vi "Untitled 1.vi"   [LabVIEW 2014]
uses:
  <vilib>/Rock Robotics/WPI/Solenoid/WPI_SolenoidValue.ctl
  <vilib>/Rock Robotics/WPI/Solenoid/WPI_SolenoidSetEnum.vi
  Robot Global Data.vi
types:
  T1 = typedef "WPI_SolenoidValue.ctl" = enum16{"Off", "On", "Forward", "Reverse"}
  T2 = typedef "WPI_SolenoidDevRef.ctl" = cluster{"DevStatus":errorcluster, "Pneumatics Control Module":u8, "Forward Solenoid Channel":T3, "Reverse Solenoid Channel":T3}
  T3 = typedef "WPI_SolenoidChannel.ctl" = enum8{"Solenoid 0", "Solenoid 1", "Solenoid 2", "Solenoid 3", "Solenoid 4", "Solenoid 5", "Solenoid 6", "Solenoid 7", "Invalid"}
  T4 = typedef "WPI_EncoderDevRef.ctl" = cluster{"DevStatus":errorcluster, "EncoderIndex":T5, "CounterIndex":T6, "DistancePerCount":dbl, "Decoding Type":T7}
  T5 = typedef "FPGA_EncoderIdx.ctl" = enum8{"Enc 0", "Enc 1", "Enc 2", "Enc 3", "Enc 4", "Enc 5", "Enc 6", "Enc 7", "Invalid"}
  T6 = typedef "FPGA_CounterCtrSystemIndex.ctl" = enum8{"Ctr 0", "Ctr 1", "Ctr 2", "Ctr 3", "Ctr 4", "Ctr 5", "Ctr 6", "Ctr 7", "Invalid"}
  T7 = typedef "WPI_EncoderType.ctl" = enum16{"1x", "2x", "4x"}
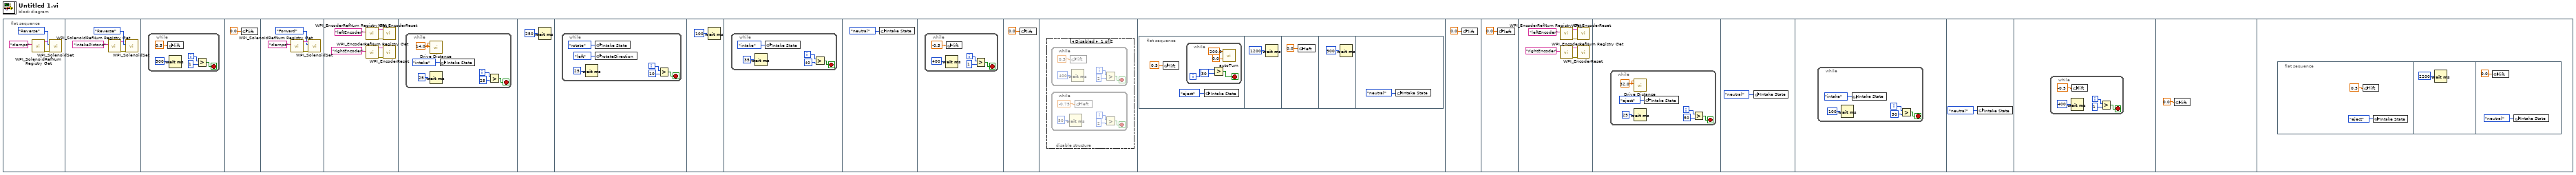
[diagram p0: block diagram]
diagram:
  n1 = flat-sequence {
    frame #0 {
      n2 = call <vilib>:"WPI_SolenoidRefNum Registry Get.vi"("refnum name"="clamps") -> ("error out"=w1:errorcluster, "SolenoidDevRef"=w2:T2)  [unwired: 9 in]
      n3 = call-poly <vilib>:"WPI_SolenoidSet.vi"("error in (no error)"=w1, "Value"=WPI_SolenoidValue."Reverse", "SolenoidDevRef"=w2) -> ()  [unwired: 7 in, 2 out]
    }
    frame #1 {
      n4 = call <vilib>:"WPI_SolenoidRefNum Registry Get.vi"("refnum name"="intakePistons") -> ("error out"=w5:errorcluster, "SolenoidDevRef"=w6:T2)  [unwired: 9 in]
      n5 = call-poly <vilib>:"WPI_SolenoidSet.vi"("error in (no error)"=w5, "Value"=WPI_SolenoidValue."Reverse", "SolenoidDevRef"=w6) -> ()  [unwired: 7 in, 2 out]
    }
    frame #2 {
      n6 = while {
        i -> [w11]
        stop <- w9 stop-if-true
        n7 = global write "Robot Global Data.vi" "lift"(0.5 ("lift")) -> ()
        n8 = Wait (ms)(milliseconds to wait=u32 500) -> ()  [unwired: 1 out]
        n9 = Greater?(x=w11, y=1) -> (0:w9:bool)
      }
    }
    frame #3 {
      n10 = global write "Robot Global Data.vi" "lift"(0.0 ("lift")) -> ()
    }
    frame #4 {
      n11 = call <vilib>:"WPI_SolenoidRefNum Registry Get.vi"("refnum name"="clamps") -> ("error out"=w18:errorcluster, "SolenoidDevRef"=w17:T2)  [unwired: 9 in]
      n12 = call-poly <vilib>:"WPI_SolenoidSet.vi"("error in (no error)"=w18, "Value"=WPI_SolenoidValue."Forward", "SolenoidDevRef"=w17) -> ()  [unwired: 7 in, 2 out]
    }
    frame #5 {
      n13 = call <vilib>:"WPI_EncoderRefNum Registry Get.vi"("refnum name"="leftEncoder") -> ("error out"=w24:errorcluster, "EncoderDevRef"=w23:T4)  [unwired: 9 in]
      n14 = call <vilib>:"WPI_EncoderRefNum Registry Get.vi"("refnum name"="rightEncoder") -> ("error out"=w19:errorcluster, "EncoderDevRef"=w20:T4)  [unwired: 9 in]
      n15 = call <vilib>:"WPI_EncoderReset.vi"("error in (no error)"=w24, "EncoderDevRef"=w23) -> ()  [unwired: 8 in, 2 out]
      n16 = call <vilib>:"WPI_EncoderReset.vi"("error in (no error)"=w19, "EncoderDevRef"=w20) -> ()  [unwired: 8 in, 2 out]
    }
    frame #6 {
      n17 = while {
        i -> [w28]
        stop <- w26 stop-if-true
        w29 = 14.0 ("Desired Right Inches")
        n18 = call "Drive Distance.vi"("Desired Right Inches"=w29, "Desired Left Inches"=w29) -> ()  [unwired: 10 in]
        n19 = Wait (ms)(milliseconds to wait=u32 25) -> ()  [unwired: 1 out]
        n20 = global write "Robot Global Data.vi" "Intake State"(enum16{"neutral", "rotate", "intake", "eject"}."intake" ("Intake State")) -> ()
        n21 = Greater?(x=w28, y=25) -> (0:w26:bool)
      }
    }
    frame #7 {
      n22 = Wait (ms)(milliseconds to wait=u32 250) -> ()  [unwired: 1 out]
    }
    frame #8 {
      n23 = while {
        i -> [w35]
        stop <- w34 stop-if-true
        n24 = Wait (ms)(milliseconds to wait=u32 25) -> ()  [unwired: 1 out]
        n25 = global write "Robot Global Data.vi" "Intake State"(enum16{"neutral", "rotate", "intake", "eject"}."rotate" ("Intake State")) -> ()
        n26 = global write "Robot Global Data.vi" "rotateDirection"(enum16{"left", "right"}."left" ("rotateDirection")) -> ()
        n27 = Greater?(x=w35, y=10) -> (0:w34:bool)
      }
    }
    frame #9 {
      n28 = Wait (ms)(milliseconds to wait=u32 100) -> ()  [unwired: 1 out]
    }
    frame #10 {
      n29 = while {
        i -> [w42]
        stop <- w41 stop-if-true
        n30 = Wait (ms)(milliseconds to wait=u32 35) -> ()  [unwired: 1 out]
        n31 = global write "Robot Global Data.vi" "Intake State"(enum16{"neutral", "rotate", "intake", "eject"}."intake" ("Intake State")) -> ()
        n32 = Greater?(x=w42, y=40) -> (0:w41:bool)
      }
    }
    frame #11 {
      n33 = global write "Robot Global Data.vi" "Intake State"(enum16{"neutral", "rotate", "intake", "eject"}."neutral" ("Intake State")) -> ()
    }
    frame #12 {
      n34 = while {
        i -> [w47]
        stop <- w45 stop-if-true
        n35 = Wait (ms)(milliseconds to wait=u32 400) -> ()  [unwired: 1 out]
        n36 = global write "Robot Global Data.vi" "lift"(-0.5 ("lift")) -> ()
        n37 = Greater?(x=w47, y=1) -> (0:w45:bool)
      }
    }
    frame #13 {
      n38 = global write "Robot Global Data.vi" "lift"(0.0 ("lift")) -> ()
    }
    frame #14 {
      n39 = disable-structure shown="Disabled" {
        frame Disabled {
          n40 = while {
            i -> [w53]
            stop <- w51 stop-if-true
            n41 = global write "Robot Global Data.vi" "lift"(0.5 ("lift")) -> ()
            n42 = Wait (ms)(milliseconds to wait=u32 400) -> ()  [unwired: 1 out]
            n43 = Greater?(x=w53, y=2) -> (0:w51:bool)
          }
          n44 = while {
            i -> [w59]
            stop <- w57 stop-if-true
            n45 = Wait (ms)(milliseconds to wait=u32 50) -> ()  [unwired: 1 out]
            n46 = global write "Robot Global Data.vi" "left"(-0.75 ("lift")) -> ()
            n47 = Greater?(x=w59, y=2) -> (0:w57:bool)
          }
        }
        frame Enabled {
        }
      }
    }
    frame #15 {
      n48 = flat-sequence {
        frame #0 {
          n49 = global write "Robot Global Data.vi" "lift"(0.5 ("lift")) -> ()
          n50 = while {
            i -> [w64]
            stop <- w65 stop-if-true
            n51 = Greater?(x=w64, y=30) -> (0:w65:bool)
            n52 = call "autoTurn.vi"("rightEncoderDesired"=0.0, "leftEncoderDesired"=200.0) -> ()  [unwired: 10 in]
          }
          n53 = global write "Robot Global Data.vi" "Intake State"(enum16{"neutral", "rotate", "intake", "eject"}."eject" ("Intake State")) -> ()
        }
        frame #1 {
          n54 = Wait (ms)(milliseconds to wait=u32 1200) -> ()  [unwired: 1 out]
        }
        frame #2 {
          n55 = global write "Robot Global Data.vi" "left"(0.0 ("lift")) -> ()
        }
        frame #3 {
          n56 = Wait (ms)(milliseconds to wait=u32 900) -> ()  [unwired: 1 out]
        }
        frame #4 {
          n57 = global write "Robot Global Data.vi" "Intake State"(enum16{"neutral", "rotate", "intake", "eject"}."neutral" ("Intake State")) -> ()
        }
      }
    }
    frame #16 {
      n58 = global write "Robot Global Data.vi" "lift"(0.0 ("lift")) -> ()
    }
    frame #17 {
      n59 = global write "Robot Global Data.vi" "left"(0.0 ("lift")) -> ()
    }
    frame #18 {
      n60 = call <vilib>:"WPI_EncoderRefNum Registry Get.vi"("refnum name"="leftEncoder") -> ("error out"=w79:errorcluster, "EncoderDevRef"=w78:T4)  [unwired: 9 in]
      n61 = call <vilib>:"WPI_EncoderRefNum Registry Get.vi"("refnum name"="rightEncoder") -> ("error out"=w74:errorcluster, "EncoderDevRef"=w75:T4)  [unwired: 9 in]
      n62 = call <vilib>:"WPI_EncoderReset.vi"("error in (no error)"=w79, "EncoderDevRef"=w78) -> ()  [unwired: 8 in, 2 out]
      n63 = call <vilib>:"WPI_EncoderReset.vi"("error in (no error)"=w74, "EncoderDevRef"=w75) -> ()  [unwired: 8 in, 2 out]
    }
    frame #19 {
      n64 = while {
        i -> [w83]
        stop <- w81 stop-if-true
        w84 = 32.0 ("Desired Right Inches")
        n65 = call "Drive Distance.vi"("Desired Right Inches"=w84, "Desired Left Inches"=w84) -> ()  [unwired: 10 in]
        n66 = Wait (ms)(milliseconds to wait=u32 25) -> ()  [unwired: 1 out]
        n67 = global write "Robot Global Data.vi" "Intake State"(enum16{"neutral", "rotate", "intake", "eject"}."eject" ("Intake State")) -> ()
        n68 = Greater?(x=w83, y=50) -> (0:w81:bool)
      }
    }
    frame #20 {
      n69 = global write "Robot Global Data.vi" "Intake State"(enum16{"neutral", "rotate", "intake", "eject"}."neutral" ("Intake State")) -> ()
    }
    frame #21 {
      n70 = while {
        i -> [w90]
        stop <- w88 stop-if-true
        n71 = Wait (ms)(milliseconds to wait=u32 100) -> ()  [unwired: 1 out]
        n72 = global write "Robot Global Data.vi" "Intake State"(enum16{"neutral", "rotate", "intake", "eject"}."intake" ("Intake State")) -> ()
        n73 = Greater?(x=w90, y=50) -> (0:w88:bool)
      }
    }
    frame #22 {
      n74 = global write "Robot Global Data.vi" "Intake State"(enum16{"neutral", "rotate", "intake", "eject"}."neutral" ("Intake State")) -> ()
    }
    frame #23 {
      n75 = while {
        i -> [w95]
        stop <- w93 stop-if-true
        n76 = Wait (ms)(milliseconds to wait=u32 400) -> ()  [unwired: 1 out]
        n77 = global write "Robot Global Data.vi" "lift"(-0.5 ("lift")) -> ()
        n78 = Greater?(x=w95, y=1) -> (0:w93:bool)
      }
    }
    frame #24 {
      n79 = global write "Robot Global Data.vi" "lift"(0.0 ("lift")) -> ()
    }
    frame #25 {
      n80 = flat-sequence {
        frame #0 {
          n81 = global write "Robot Global Data.vi" "lift"(0.5 ("lift")) -> ()
          n82 = global write "Robot Global Data.vi" "Intake State"(enum16{"neutral", "rotate", "intake", "eject"}."eject" ("Intake State")) -> ()
        }
        frame #1 {
          n83 = Wait (ms)(milliseconds to wait=u32 2200) -> ()  [unwired: 1 out]
        }
        frame #2 {
          n84 = global write "Robot Global Data.vi" "lift"(0.0 ("lift")) -> ()
          n85 = global write "Robot Global Data.vi" "Intake State"(enum16{"neutral", "rotate", "intake", "eject"}."neutral" ("Intake State")) -> ()
        }
      }
    }
  }
